vi "Dialog_Enter Generic.vi"(8 "Error In":errorcluster, 11 "Parameter Table":string[][](array[string])) -> (0 "Error Out":errorcluster, 2 "Cancelled?":bool, 3 "Generic Command":string)   [LabVIEW 2012]
doc: "SciScan 1.2 160622\nThis is the dialog box which pops up when teh user wants to enter a generic Macro command"
uses:
  CustomControls/DataTypeSelector.ctl
  Custom Controls and Typedefs/Delete Button.ctl
  Custom Controls and Typedefs/BOOL Enum.ctl
  Dialog Enter Generic_UICtrlRefnums.ctl
  <vilib>/Utility/VariantDataType/Type.ctl
  CommonResource VIs/UI Control and Indicator properties_Commands.ctl
  SubVIs/UpdateDialogWithGFGValue_Command.ctl
  <vilib>/Utility/VariantDataType/VariantType.lvlib
panel:
  out "Current BOOL Value":T1
  in  "Enter BOOL Value":T1
  in  "Delete":T2
  out "Current Path Value":path
  out "Current String Value":string
  out "Current Numeric Value":dbl
  in  "Use current":bool
  in  "Data Type":T3
  in  "Parameters":i32(listbox)
  in  "Add":bool
  in  "Enter Path Value":path
  in  "Enter String Value":string
  in  "Enter Numeric Value":dbl
  in  "Cancel Button":bool
  in  "OK Button":bool
  in  "GFG Variable Name":string(combo)
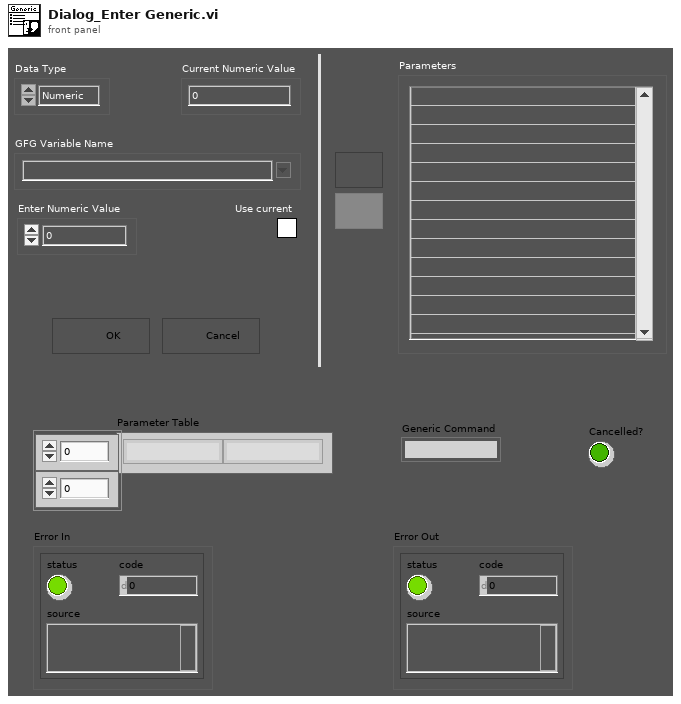
[diagram p1: front panel]
types:
  T1 = typedef "BOOL Enum.ctl" = enum16{"FALSE", "TRUE"}
  T2 = typedef "Delete Button.ctl" = bool
  T3 = typedef "DataTypeSelector.ctl" = enum16{"Numeric", "Boolean", "String", "Path"}
  T4 = typedef "VariantType.lvlib/Type.ctl" = enum8{"Invalid Type", "Void", "I8", "I16", "I32", "I64", "U8", "U16", "U32", "U64", "Single Float", "Double Float", "Extended Float", "Single Complex", "Double Complex", "Extended Complex", "Enum U8", "Enum U16", "Enum U32", "Enum U64", "Single Float With Unit", "Double Float With Unit", "Extended Float With Unit", "Single Complex with Unit", "Double Complex with Unit", "Extended Complex with Unit", "Boolean", "String", "Path", "Picture", "Tag", "Array", "Cluster", "Variant", "LV Variant", "Waveform", "Timestamp", "Digital Waveform", "Digital Data", "ExpressData", "Refnum", "External Data", "VI", "Poly VI", "LabVIEW Class Instance", "Fixed Point"}
  T5 = typedef "Dialog Enter Generic_UICtrlRefnums.ctl" = cluster{"Enter Numeric Value":refnum<vi>, "Enter BOOL Value":refnum<vi>, "Enter String Value":refnum<vi>, "Enter Path Value":refnum<vi>, "Add":refnum<vi>, "Data Type":refnum<vi>, "Parameters":refnum<vi>, "GFG Variable Name":refnum<vi>, "OK Button":refnum<vi>, "Current Numeric Value":refnum<vi>, "Current BOOL Value":refnum<vi>, "Current String Value":refnum<vi>, "Current Path Value":refnum<vi>, "UseCurrent Checkbox":refnum<vi>, "Delete":refnum<vi>}
  T6 = enum8{"Enabled", "Disabled", "Disabled and Grayed Out"}
  T7 = typedef "UI Control and Indicator properties_Commands.ctl" = enum16{"Enable", "Disable", "Disable and Grey", "Make Visible", "Make Invisible"}
  T8 = typedef "UpdateDialogWithGFGValue_Command.ctl" = enum16{"Update", "Invalidate"}
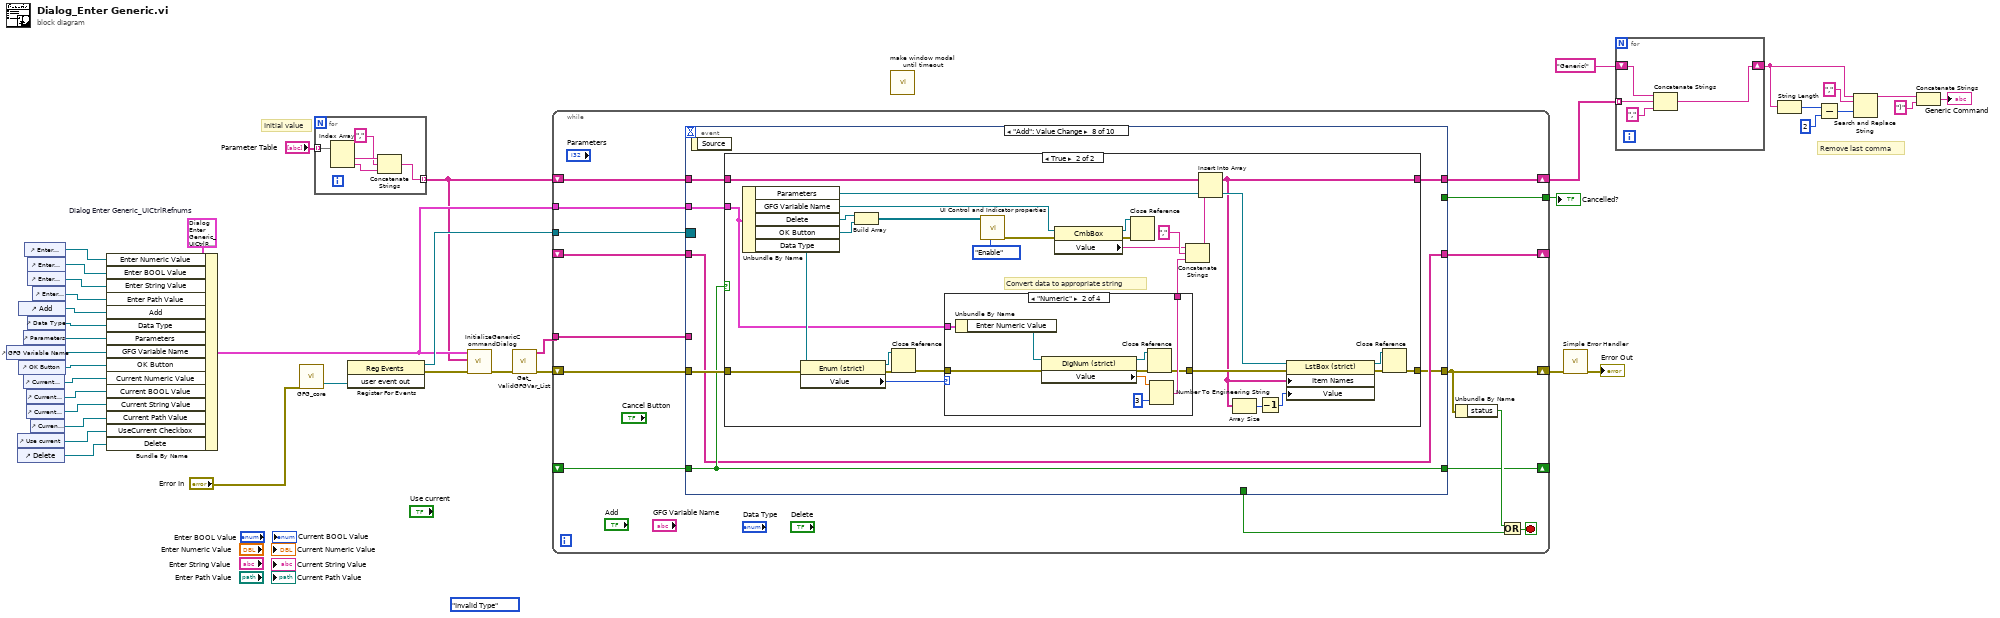
[diagram p0: block diagram]
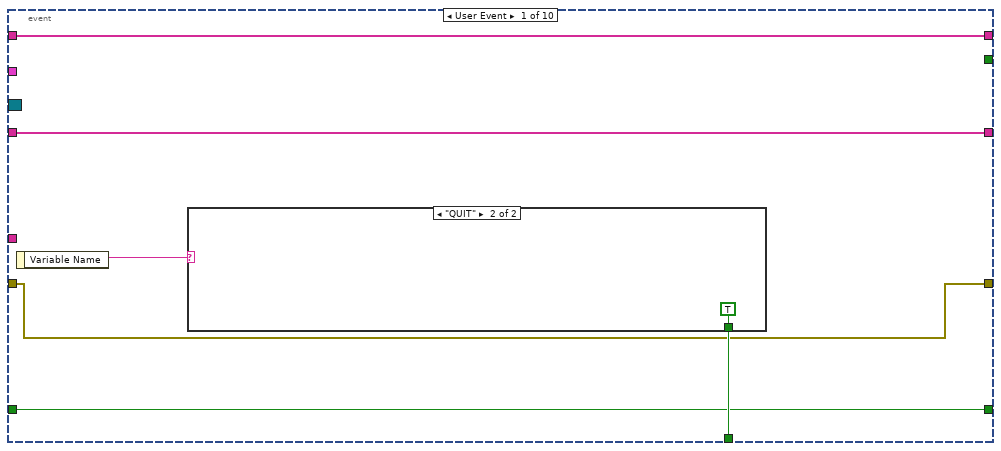
[diagram p2: hidden frame]
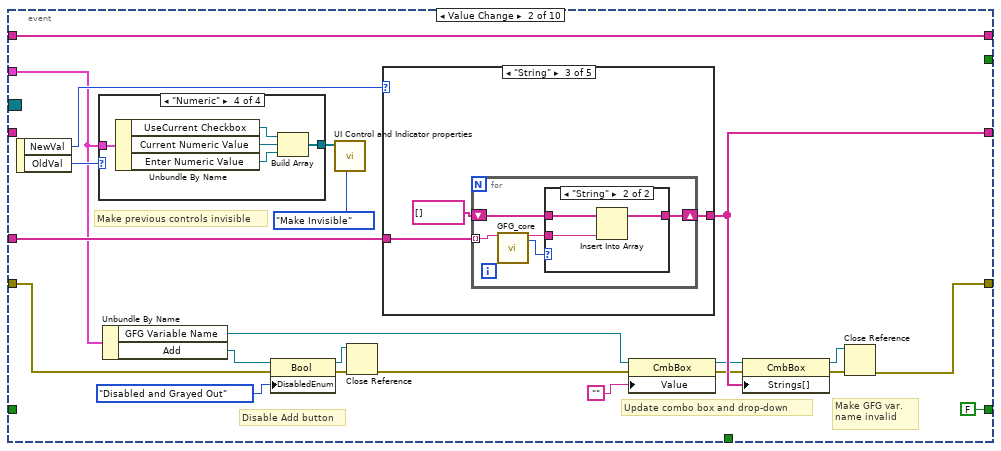
[diagram p4: hidden frame]
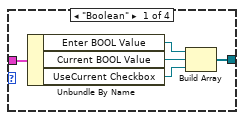
[diagram p5: hidden frame]
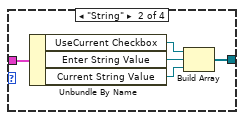
[diagram p6: hidden frame]
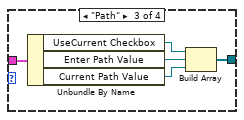
[diagram p7: hidden frame]
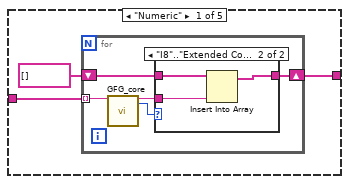
[diagram p8: hidden frame]
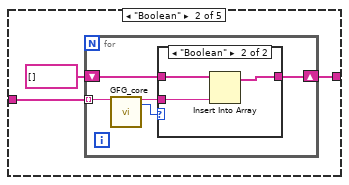
[diagram p10: hidden frame]
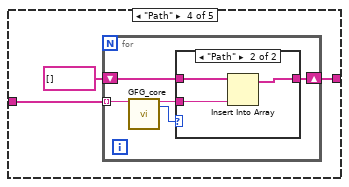
[diagram p13: hidden frame]
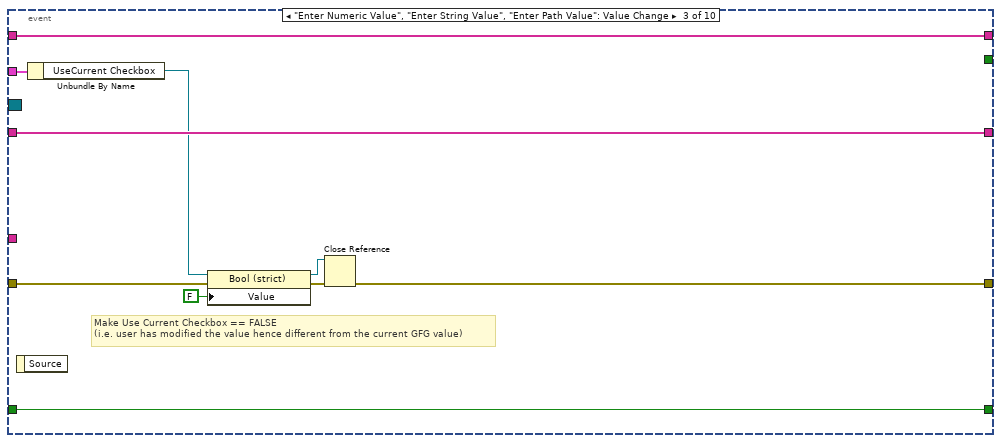
[diagram p16: hidden frame]
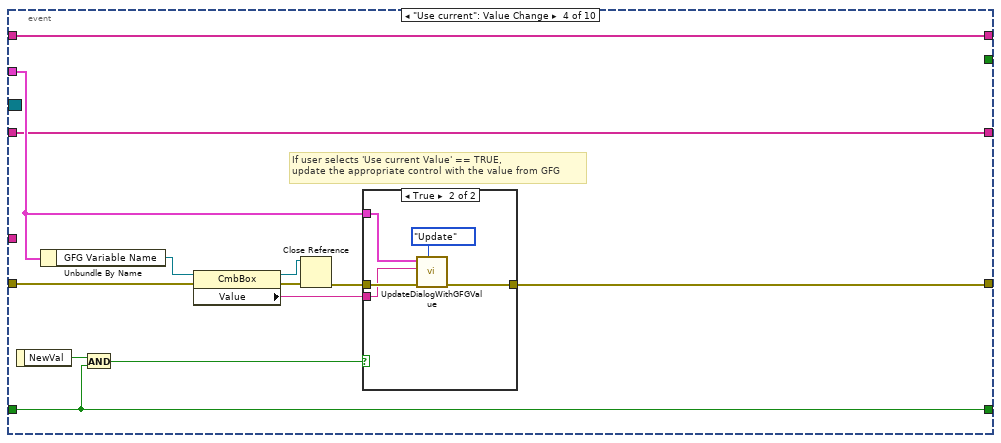
[diagram p17: hidden frame]
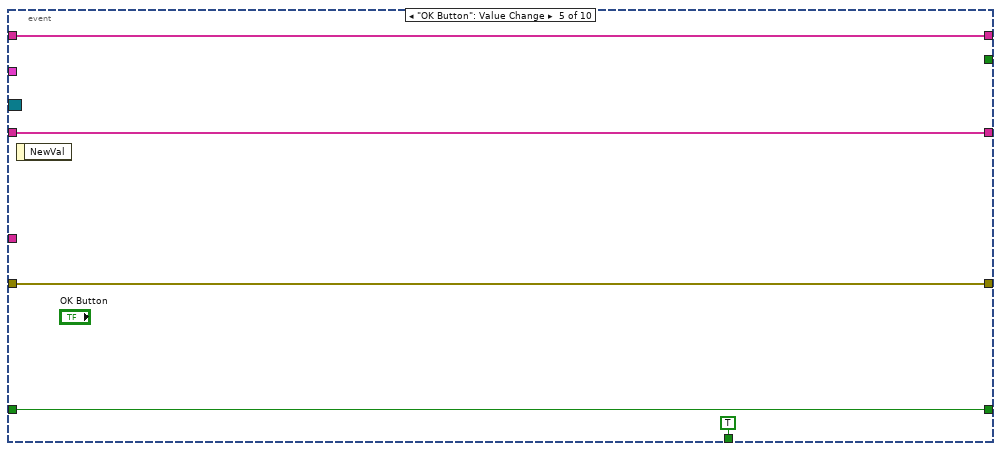
[diagram p19: hidden frame]
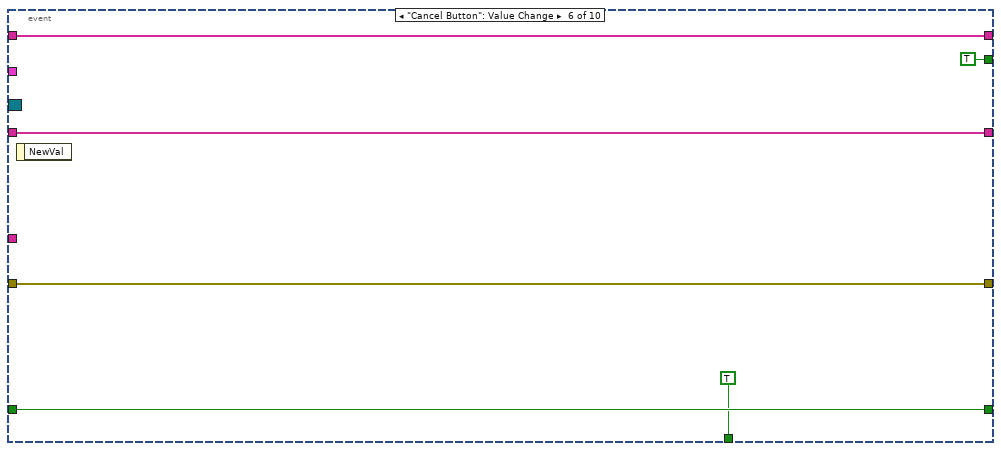
[diagram p20: hidden frame]
diagram:
  (unwired) Type."Invalid Type" ("Data Type Out")
  w36 = T5 {"Enter Numeric Value"=refnum, "Enter BOOL Value"=refnum, "Enter String Value"=refnum, "Enter Path Value"=refnum, "Add"=refnum, "Data Type"=refnum, "Parameters"=refnum, "GFG Variable Name"=refnum, "OK Button"=refnum, "Current Numeric Value"=refnum, "Current BOOL Value"=refnum, "Current String Value"=refnum, "Current Path Value"=refnum, "UseCurrent Checkbox"=refnum, "Delete"=refnum}  # Dialog Enter Generic_UICtrlRefnums
  # "Initial value"
  # "Remove last comma"
  n1 = control-ref of="GFG Variable Name"() -> (w35:refnum<vi>)
  n2 = control-ref of="Use current"() -> (w20:refnum<vi>)
  n3 = control-ref of="Delete"() -> (w19:refnum<vi>)
  n4 = control-ref of="Add"() -> (w33:refnum<vi>)
  n5 = control-ref of="OK Button"() -> (w26:refnum<vi>)
  n6 = control-ref of="Parameters"() -> (w34:refnum<vi>)
  n7 = control-ref of="Current Numeric Value"() -> (w25:refnum<vi>)
  n8 = control-ref of="Enter Numeric Value"() -> (w30:refnum<vi>)
  n9 = control-ref of="Current BOOL Value"() -> (w21:refnum<vi>)
  n10 = control-ref of="Current String Value"() -> (w24:refnum<vi>)
  n11 = control-ref of="Enter BOOL Value"() -> (w22:refnum<vi>)
  n12 = control-ref of="Enter String Value"() -> (w31:refnum<vi>)
  n13 = control-ref of="Data Type"() -> (w29:refnum<vi>)
  n14 = control-ref of="Current Path Value"() -> (w23:refnum<vi>)
  n15 = control-ref of="Enter Path Value"() -> (w32:refnum<vi>)
  n16 = Bundle By Name(cluster=w36, "Enter Numeric Value"=w30, "Enter BOOL Value"=w22, "Enter String Value"=w31, "Enter Path Value"=w32, "Add"=w33, "Data Type"=w29, "Parameters"=w34, "GFG Variable Name"=w35, "OK Button"=w26, "Current Numeric Value"=w25, "Current BOOL Value"=w21, "Current String Value"=w24, "Current Path Value"=w23, "UseCurrent Checkbox"=w20, "Delete"=w19) -> (w17:T5)
  n17 = call "GFG_core.vi"("error in (no error)"="Error In") -> ("user event out"=w39:refnum<user-event>)  [unwired: 12 in, 6 out]
  n18 = for {
    tunnel: "Parameter Table" -> [w44] mode=indexing
    tunnel: [w40] -> w1 mode=indexing
    n19 = Index Array(array=w44) -> (element #1=w43:string, element #2=w41:string)  [unwired: 2 in]
    n20 = Concatenate Strings(w43, "," ("string"), w41) -> (w40:string)
  }
  n21 = register-events(w39) -> (reference out=w38:refnum<event-registration>, error out=w18:errorcluster)  [unwired: 2 in]
  n22 = call "InitializeGenericCommandDialog.vi"("Error In"=w18, "Initial List Values"=w1, "Dialog Enter Generic_UICtrlRefnums"=w17) -> ("Error Out"=w16:errorcluster)  [unwired: 8 in]
  n23 = call "Get_ValidGFGVar_List.vi"("Error In"=w16) -> ("Error Out"=w14:errorcluster, "All Variable Names Out"=w15:string[])  [unwired: 9 in]
  n24 = while {
    tunnel: w38 -> [w59]
    shift-right: [w53] -> w28
    shift-left: w14 -> [w58]
    tunnel: w15 -> [w57]
    tunnel: w17 -> [w56]
    shift-right: [w55] -> _
    shift-left: _ -> [w54]
    shift-right: [w49] -> _
    shift-left: _ -> [w48]
    shift-right: [w46] -> w12
    shift-left: w1 -> [w47]
    tunnel: [w45] -> w13
    stop <- w50 stop-if-true
    n25 = event shown="[7] \"Add\": Value Change" {
      selector: w59 -> [_ _ _ _ _ _ _ _ _ _]
      dyn-events: _ -> [_ _ _ _ _ _ _ _ _ _]
      timeout: _ -> [_ _ _ _ _ _ _ _ _ _]
      tunnel: [w64 _ _ _ TRUE TRUE _ _ _ TRUE] -> w51
      tunnel: [w63 w71 w160 w170 w190 w197 w200 w252 w330 w374] -> w53
      tunnel: w58 -> [w63 w70 w164 w177 w190 w197 w211 w257 w334 w374]
      tunnel: w57 -> [_ w87 _ _ _ _ _ _ _ _]
      tunnel: w56 -> [_ w80 w166 w171 _ _ w201 w253 w331 _]
      tunnel: [w62 w84 w167 w169 w189 w194 w208 w254 w332 w372] -> w55
      tunnel: w54 -> [w62 _ w167 w169 w189 w194 w208 w254 w332 w372]
      tunnel: [w61 FALSE w159 w179 w188 w193 w199 w255 w333 w371] -> w49
      tunnel: w48 -> [w61 _ w159 w179 w188 w193 _ w255 w333 w371]
      tunnel: w47 -> [w60 w67 w158 w168 w187 w195 w198 w256 w328 w373]
      tunnel: [w60 w67 w158 w168 w187 w195 w198 w251 w329 w373] -> w46
      tunnel: [_ _ _ _ _ TRUE _ _ _ TRUE] -> w45
      event User Event {
        n26 = event-data() -> ("Variable Name"=w65:string)  [unwired: 1 in]
        n27 = case shown="\"QUIT\"" w65 {
          tunnel: [_ TRUE] -> w64
          frame Default {
          }
          frame "QUIT" {
          }
        }
      }
      event Value Change {
        # "Disable Add button"
        # "Update combo box and drop-down"
        # "Make GFG var. name invalid"
        # "Make previous controls invisible"
        n28 = event-data() -> ("NewVal"=w88:T3, "OldVal"=w81:T3)  [unwired: 1 in]
        n29 = case shown="\"Numeric\"" w81 {
          tunnel: w80 -> [w93 w98 w103 w108]
          tunnel: [w90 w95 w100 w105] -> w78
          frame "Boolean" {
            n30 = Unbundle By Name(w93) -> ("Enter BOOL Value"=w91:refnum<vi>, "Current BOOL Value"=w92:refnum<vi>, "UseCurrent Checkbox"=w89:refnum<vi>)
            n31 = Build Array(w91, w92, w89) -> (w90:refnum<vi>[])
          }
          frame "String" {
            n32 = Unbundle By Name(w98) -> ("UseCurrent Checkbox"=w94:refnum<vi>, "Enter String Value"=w96:refnum<vi>, "Current String Value"=w97:refnum<vi>)
            n33 = Build Array(w94, w96, w97) -> (w95:refnum<vi>[])
          }
          frame "Path" {
            n34 = Unbundle By Name(w103) -> ("UseCurrent Checkbox"=w99:refnum<vi>, "Enter Path Value"=w101:refnum<vi>, "Current Path Value"=w102:refnum<vi>)
            n35 = Build Array(w99, w101, w102) -> (w100:refnum<vi>[])
          }
          frame "Numeric" {
            n36 = Unbundle By Name(w108) -> ("UseCurrent Checkbox"=w104:refnum<vi>, "Current Numeric Value"=w106:refnum<vi>, "Enter Numeric Value"=w107:refnum<vi>)
            n37 = Build Array(w104, w106, w107) -> (w105:refnum<vi>[])
          }
        }
        n38 = Unbundle By Name(w80) -> ("GFG Variable Name"=w85:refnum<vi>, "Add"=w69:refnum<vi>)
        n39 = property class="Bool"(reference=w69, error in=w70, "DisabledEnum"=T6."Disabled and Grayed Out" ("Disabled")) -> (reference out=w75:refnum<vi>, error out=w76:errorcluster)
        n40 = call "UI Control and Indicator properties.vi"("Enable Command"=UI_Control_and_Indicator_properties_Commands."Make Invisible", "Control Refnums"=w78) -> ()  [unwired: 9 in, 1 out]
        n41 = Close Reference(reference=w75, error in (no error)=w76) -> (error out=w68:errorcluster)
        n42 = case shown="\"String\"" w88 {
          tunnel: w87 -> [w111 w123 w135 w147 w157]
          tunnel: [w109 w121 w133 w145 w157] -> w84
          frame "Numeric" {
            n43 = for {
              tunnel: w111 -> [w116] mode=indexing
              shift-right: [w112] -> w109
              shift-left: string[] [] ("All Variable Names Out") -> [w113]
              n44 = call "GFG_core.vi"("Variable Name in"=w116) -> ("Variable Name Out"=w114:string, "Data Type Out"=w115:T4)  [unwired: 12 in, 5 out]
              n45 = case shown="\"I8\"..\"Extended Complex\"" w115 {
                tunnel: w114 -> [_ w119]
                tunnel: w113 -> [w117 w120]
                tunnel: [w117 w118] -> w112
                frame Default {
                }
                frame "I8".."Extended Complex" {
                  n46 = Insert Into Array(array=w120, new element=w119) -> (w118:string[])  [unwired: 1 in]
                }
              }
            }
          }
          frame "Boolean" {
            n47 = for {
              tunnel: w123 -> [w128] mode=indexing
              shift-right: [w124] -> w121
              shift-left: string[] [] ("All Variable Names Out") -> [w125]
              n48 = call "GFG_core.vi"("Variable Name in"=w128) -> ("Variable Name Out"=w126:string, "Data Type Out"=w127:T4)  [unwired: 12 in, 5 out]
              n49 = case shown="\"Boolean\"" w127 {
                tunnel: w126 -> [_ w131]
                tunnel: w125 -> [w129 w132]
                tunnel: [w129 w130] -> w124
                frame Default {
                }
                frame "Boolean" {
                  n50 = Insert Into Array(array=w132, new element=w131) -> (w130:string[])  [unwired: 1 in]
                }
              }
            }
          }
          frame "String" {
            n51 = for {
              tunnel: w135 -> [w140] mode=indexing
              shift-right: [w136] -> w133
              shift-left: string[] [] ("All Variable Names Out") -> [w137]
              n52 = call "GFG_core.vi"("Variable Name in"=w140) -> ("Variable Name Out"=w138:string, "Data Type Out"=w139:T4)  [unwired: 12 in, 5 out]
              n53 = case shown="\"String\"" w139 {
                tunnel: w138 -> [_ w143]
                tunnel: w137 -> [w141 w144]
                tunnel: [w141 w142] -> w136
                frame Default {
                }
                frame "String" {
                  n54 = Insert Into Array(array=w144, new element=w143) -> (w142:string[])  [unwired: 1 in]
                }
              }
            }
          }
          frame "Path" {
            n55 = for {
              tunnel: w147 -> [w152] mode=indexing
              shift-right: [w148] -> w145
              shift-left: string[] [] ("All Variable Names Out") -> [w149]
              n56 = call "GFG_core.vi"("Variable Name in"=w152) -> ("Variable Name Out"=w150:string, "Data Type Out"=w151:T4)  [unwired: 12 in, 5 out]
              n57 = case shown="\"Path\"" w151 {
                tunnel: w150 -> [_ w155]
                tunnel: w149 -> [w153 w156]
                tunnel: [w153 w154] -> w148
                frame Default {
                }
                frame "Path" {
                  n58 = Insert Into Array(array=w156, new element=w155) -> (w154:string[])  [unwired: 1 in]
                }
              }
            }
          }
          frame Default {
          }
        }
        n59 = property class="CmbBox"(reference=w85, error in=w68, "Value"="") -> (reference out=w83:refnum<vi>, error out=w82:errorcluster)
        n60 = property class="CmbBox"(reference=w83, error in=w82, "Strings[]"=w84) -> (reference out=w72:refnum<vi>, error out=w73:errorcluster)
        n61 = Close Reference(reference=w72, error in (no error)=w73) -> (error out=w71:errorcluster)
      }
      event "Enter Numeric Value", "Enter String Value", "Enter Path Value": Value Change {
        # "Make Use Current Checkbox == FALSE\n(i.e. user has modified the value hence different from the current GFG value)"
        n62 = event-data() -> ()  [unwired: 1 in, 1 out]
        n63 = Unbundle By Name(w166) -> ("UseCurrent Checkbox"=w165:refnum<vi>)
        n64 = property class="Bool (strict)"(reference=w165, error in=w164, "Value"=FALSE) -> (reference out=w161:refnum<vi>, error out=w162:errorcluster)
        n65 = Close Reference(reference=w161, error in (no error)=w162) -> (error out=w160:errorcluster)
      }
      event "Use current": Value Change {
        # "If user selects 'Use current Value' == TRUE,\nupdate the appropriate control with the value from GFG"
        n66 = event-data() -> ("NewVal"=w180:bool)  [unwired: 1 in]
        n67 = Unbundle By Name(w171) -> ("GFG Variable Name"=w178:refnum<vi>)
        n68 = And(x=w180, y=w179) -> (x .and. y?=w174:bool)
        n69 = property class="CmbBox"(reference=w178, error in=w177) -> (reference out=w175:refnum<vi>, error out=w176:errorcluster, "Value"=w173:string)
        n70 = Close Reference(reference=w175, error in (no error)=w176) -> (error out=w172:errorcluster)
        n71 = case shown="True" w174 {
          tunnel: w173 -> [_ w184]
          tunnel: w172 -> [w181 w185]
          tunnel: w171 -> [_ w183]
          tunnel: [w181 w182] -> w170
          frame False {
          }
          frame True {
            n72 = call "UpdateDialogWithGFGValue.vi"("UpdateDialogWithGFGValue_Comamnd"=UpdateDialogWithGFGValue_Command."Update", "Error In"=w185, "Variable Name"=w184, "Dialog Enter Generic_UICtrlRefnums"=w183) -> ("Error Out"=w182:errorcluster)  [unwired: 7 in]
          }
        }
      }
      event "OK Button": Value Change {
        n73 = event-data() -> ()  [unwired: 1 in, 1 out]
      }
      event "Cancel Button": Value Change {
        n74 = event-data() -> ()  [unwired: 1 in, 1 out]
      }
      event "GFG Variable Name": Value Change {
        # "1. Update the drop-down string list based on user entered string value\n2. Check if a valid GFG variable name has been entered/selected"
        # "If valid variable name entered by user, fetch \ncurrent GFG value, and enable 'Add' button"
        n75 = event-data() -> ("NewVal"=w209:string)  [unwired: 1 in]
        n76 = Empty String/Path?(string/path=w209) -> (empty?=w210:bool)
        n77 = case shown="False" w210 {
          tunnel: w208 -> [w235 w250]
          tunnel: [w236 w250] -> w206
          tunnel: w209 -> [w234 _]
          tunnel: [w232 FALSE] -> w199
          frame False {
            n78 = Search 1D Array(1D array=w235, element=w234) -> (index of element=w233:i32)  [unwired: 1 in]
            n79 = Greater Or Equal To 0?(x=w233) -> (x >= 0?=w232:bool)
            n80 = for {
              tunnel: w235 -> [w241] mode=indexing
              tunnel: w234 -> [w238]
              shift-right: [w243] -> w236
              shift-left: string[] [] -> [w244]
              n81 = Search and Replace String(case sensitive?=TRUE ("ignore case? (F)"), input string=w241, search string=w238) -> (number of replacements=w240:i32)  [unwired: 5 in, 3 out]
              n82 = Greater Than 0?(x=w240) -> (x > 0?=w239:bool)
              n83 = case shown="True" w239 {
                tunnel: w244 -> [w245 w248]
                tunnel: w241 -> [_ w247]
                tunnel: [w245 w246] -> w243
                frame False {
                }
                frame True {
                  n84 = Insert Into Array(array=w248, new element=w247) -> (w246:string[])  [unwired: 1 in]
                }
              }
            }
          }
          frame True {
          }
        }
        n85 = Unbundle By Name(w201) -> ("GFG Variable Name"=w207:refnum<vi>)
        n86 = property class="CmbBox"(reference=w207, error in=w211, "Strings[]"=w206) -> (reference out=w203:refnum<vi>, error out=w204:errorcluster)
        n87 = Index Array(array=w206) -> (element=w205:string)  [unwired: 1 in]
        n88 = Close Reference(reference=w203, error in (no error)=w204) -> (error out=w202:errorcluster)
        n89 = case shown="True" w199 {
          tunnel: w205 -> [w220 w230]
          tunnel: w202 -> [w221 w231]
          tunnel: w201 -> [w218 w223]
          tunnel: [w212 w225] -> w200
          frame True {
            n90 = Unbundle By Name(w218) -> ("Add"=w217:refnum<vi>)
            n91 = call "UpdateDialogWithGFGValue.vi"("UpdateDialogWithGFGValue_Comamnd"=UpdateDialogWithGFGValue_Command."Update", "Error In"=w221, "Variable Name"=w220, "Dialog Enter Generic_UICtrlRefnums"=w218) -> ("Error Out"=w215:errorcluster)  [unwired: 7 in]
            n92 = property class="Bool"(reference=w217, error in=w215, "DisabledEnum"=T6."Enabled" ("Disabled")) -> (reference out=w213:refnum<vi>, error out=w214:errorcluster)
            n93 = Close Reference(reference=w213, error in (no error)=w214) -> (error out=w212:errorcluster)
          }
          frame False {
            n94 = call "UpdateDialogWithGFGValue.vi"("UpdateDialogWithGFGValue_Comamnd"=UpdateDialogWithGFGValue_Command."Invalidate", "Error In"=w231, "Variable Name"=w230, "Dialog Enter Generic_UICtrlRefnums"=w223) -> ("Error Out"=w226:errorcluster)  [unwired: 7 in]
            n95 = Unbundle By Name(w223) -> ("Add"=w222:refnum<vi>)
            n96 = property class="Bool"(reference=w222, error in=w226, "DisabledEnum"=T6."Disabled and Grayed Out" ("Disabled")) -> (reference out=w227:refnum<vi>, error out=w228:errorcluster)
            n97 = Close Reference(reference=w227, error in (no error)=w228) -> (error out=w225:errorcluster)
          }
        }
      }
      event "Add": Value Change {
        n98 = event-data() -> ()  [unwired: 1 in, 1 out]
        n99 = case shown="True" w255 {
          tunnel: w257 -> [w258 w287]
          tunnel: w256 -> [w259 w281]
          tunnel: w253 -> [_ w273]
          tunnel: [w258 w277] -> w252
          tunnel: [w259 w268] -> w251
          frame False {
            # "INvalid GFG variable name... Don't Add!"
          }
          frame True {
            # "Convert data to appropriate string"
            n100 = Unbundle By Name(w273) -> ("Parameters"=w275:refnum<vi>, "GFG Variable Name"=w272:refnum<vi>, "Delete"=w264:refnum<vi>, "OK Button"=w263:refnum<vi>, "Data Type"=w274:refnum<vi>)
            n101 = property class="Enum (strict)"(reference=w274, error in=w287) -> (reference out=w284:refnum<vi>, error out=w285:errorcluster, "Value"=w286:enum16{"Numeric", "Boolean", "String", "Path"})
            n102 = Build Array(w264, w263) -> (w262:refnum<vi>[])
            n103 = Close Reference(reference=w284, error in (no error)=w285) -> (error out=w260:errorcluster)
            n104 = case shown="\"Numeric\"" w286 {
              tunnel: w273 -> [w296 w305 w314 w325]
              tunnel: w260 -> [w294 w303 w312 w323]
              tunnel: [w292 w300 w306 w316] -> w282
              tunnel: [w291 w298 w309 w321] -> w276
              frame "Boolean" {
                n105 = Unbundle By Name(w296) -> ("Enter BOOL Value"=w295:refnum<vi>)
                n106 = property class="Enum (strict)"(reference=w295, error in=w294) -> (reference out=w289:refnum<vi>, error out=w290:errorcluster, "Value"=w293:T1)
                n107 = Close Reference(reference=w289, error in (no error)=w290) -> (error out=w288:errorcluster)
                n108 = Format Into String(error in=w288, w293) -> (resulting string=w292:string, error out=w291:errorcluster)  [unwired: 2 in]
              }
              frame "Numeric" {
                n109 = Unbundle By Name(w305) -> ("Enter Numeric Value"=w304:refnum<vi>)
                n110 = property class="DigNum (strict)"(reference=w304, error in=w303) -> (reference out=w301:refnum<vi>, error out=w302:errorcluster, "Value"=w299:dbl)
                n111 = Close Reference(reference=w301, error in (no error)=w302) -> (error out=w298:errorcluster)
                n112 = Number To Engineering String(2:i16 3 ("precision (6)"), 4:w299) -> (0:w300:string)  [unwired: 2 in]
              }
              frame "String" {
                w307 = "'" ("string")
                n113 = Unbundle By Name(w314) -> ("Enter String Value"=w313:refnum<vi>)
                n114 = property class="Str"(reference=w313, error in=w312) -> (reference out=w310:refnum<vi>, error out=w311:errorcluster, "Value"=w308:string)
                n115 = Close Reference(reference=w310, error in (no error)=w311) -> (error out=w309:errorcluster)
                n116 = Concatenate Strings(w307, w308, w307) -> (w306:string)
              }
              frame "Path" {
                w317 = "'" ("string")
                n117 = Unbundle By Name(w325) -> ("Enter Path Value"=w324:refnum<vi>)
                n118 = property class="Path"(reference=w324, error in=w323) -> (reference out=w319:refnum<vi>, error out=w320:errorcluster, "Value"=w322:path)
                n119 = Close Reference(reference=w319, error in (no error)=w320) -> (error out=w318:errorcluster)
                n120 = Format Into String(error in=w318, w322) -> (resulting string=w315:string, error out=w321:errorcluster)  [unwired: 2 in]
                n121 = Concatenate Strings(w317, w315, w317) -> (w316:string)
              }
            }
            n122 = call "UI Control and Indicator properties.vi"("Enable Command"=UI_Control_and_Indicator_properties_Commands."Enable", "Control Refnums"=w262) -> ("Error Out"=w261:errorcluster)  [unwired: 9 in]
            n123 = property class="CmbBox"(reference=w272, error in=w261) -> (reference out=w270:refnum<vi>, error out=w271:errorcluster, "Value"=w269:string)
            n124 = Close Reference(reference=w270, error in (no error)=w271) -> ()  [unwired: 1 out]
            n125 = Concatenate Strings(w269, "," ("string"), w282) -> (w280:string)
            n126 = Insert Into Array(array=w281, new element=w280) -> (w268:string[])  [unwired: 1 in]
            n127 = Array Size(array=w268) -> (size(s)=w267:i32)
            n128 = Decrement(x=w267) -> (x-1=w266:i32)
            n129 = property class="LstBox (strict)"(reference=w275, error in=w276, "Item Names"=w268, "Value"=w266) -> (reference out=w278:refnum<vi>, error out=w279:errorcluster)
            n130 = Close Reference(reference=w278, error in (no error)=w279) -> (error out=w277:errorcluster)
          }
        }
      }
      event Value Change {
        # "Any items to delete"
        n131 = event-data() -> ()  [unwired: 1 in, 1 out]
        n132 = Array Size(array=w328) -> (size(s)=w327:i32)
        n133 = Greater Than 0?(x=w327) -> (x > 0?=w326:bool)
        n134 = case shown="True" w326 {
          tunnel: w334 -> [w336 w357]
          tunnel: w328 -> [w342 w356]
          tunnel: w331 -> [w340 w358]
          tunnel: [w335 w360] -> w330
          tunnel: [w342 w347] -> w329
          frame False {
            n135 = Unbundle By Name(w340) -> ("Delete"=w339:refnum<vi>, "OK Button"=w338:refnum<vi>)
            n136 = Build Array(w339, w338) -> (w337:refnum<vi>[])
            n137 = call "UI Control and Indicator properties.vi"("Enable Command"=UI_Control_and_Indicator_properties_Commands."Disable and Grey", "Error In"=w336, "Control Refnums"=w337) -> ("Error Out"=w335:errorcluster)  [unwired: 8 in]
          }
          frame True {
            n138 = Unbundle By Name(w358) -> ("Parameters"=w359:refnum<vi>, "Delete"=w345:refnum<vi>, "OK Button"=w344:refnum<vi>)
            n139 = property class="LstBox (strict)"(reference=w359, error in=w357) -> (reference out=w353:refnum<vi>, error out=w354:errorcluster, "Value"=w350:i32)
            n140 = Build Array(w345, w344) -> (w343:refnum<vi>[])
            n141 = Delete From Array(array=w356, length=1, index=w350) -> (array with subset deleted=w347:string[])  [unwired: 1 out]
            n142 = Array Size(array=w347) -> (size(s)=w348:i32)
            n143 = Equal To 0?(x=w348) -> (x = 0?=w346:bool)
            n144 = case shown="False" w346 {
              tunnel: w350 -> [w364 _]
              tunnel: [w361 -1 ("f")] -> w349
              tunnel: w343 -> [_ w367]
              frame False {
                # "Don't make index = -1\nif there are any elements"
                n145 = Equal To 0?(x=w364) -> (x = 0?=w365:bool)
                n146 = Decrement(x=w364) -> (x-1=w363:i32)
                n147 = Select(t=0 ("f"), s=w365, f=w363) -> (s? t:f=w361:i32)
              }
              frame True {
                n148 = call "UI Control and Indicator properties.vi"("Enable Command"=UI_Control_and_Indicator_properties_Commands."Disable and Grey", "Control Refnums"=w367) -> ()  [unwired: 9 in, 1 out]
              }
            }
            n149 = property class="LstBox (strict)"(reference=w353, error in=w354, "Item Names"=w347, "Value"=w349) -> (reference out=w351:refnum<vi>, error out=w352:errorcluster)
            n150 = Close Reference(reference=w351, error in (no error)=w352) -> (error out=w360:errorcluster)
          }
        }
      }
      event Panel Close {
        n151 = event-data() -> ()  [unwired: 1 in, 1 out]
      }
    }
    n152 = Unbundle By Name(w53) -> ("status"=w52:bool)
    n153 = Or(x=w52, y=w51) -> (x .or. y?=w50:bool)
  }
  "Cancelled?" <- w13
  n154 = call "make window modal until timeout.vi"() -> ()  [unwired: 12 in]
  n155 = call <vilib>:"Simple Error Handler.vi"("error in (no error)"=w28) -> ("error out"=→"Error Out":errorcluster)  [unwired: 4 in, 4 out]
  n156 = for {
    tunnel: w12 -> [w378] mode=indexing
    shift-right: [w376] -> w8
    shift-left: "Generic(" -> [w375]
    n157 = Concatenate Strings(w375, w378, ",") -> (w376:string)
  }
  n158 = String Length(string=w8) -> (length=w10:i32)
  n159 = Subtract(x=w10, y=2) -> (x-y=w7:i32)
  n160 = Search and Replace String(input string=w8, search string=",", offset=w7) -> (result string=w5:string)  [unwired: 5 in, 3 out]
  n161 = Concatenate Strings(w5, ")") -> (→"Generic Command":string)
